vi "Stop HTTP.vi"(8 "error in (no error)":errorcluster, 11 "Vecto in":refnum<class "Vecto.lvclass">) -> (0 "error out":errorcluster, 3 "Vecto out":refnum<class "Vecto.lvclass">)   [LabVIEW 2020, in "Vecto.lvlib" / "Vecto.lvclass"]
uses:
  Vecto.lvclass
  Vecto.lvclass/Vecto.ctl
  lv-http-server/HTTP Server/Server/Server.lvclass
  VectoService/VectoInfo.lvclass
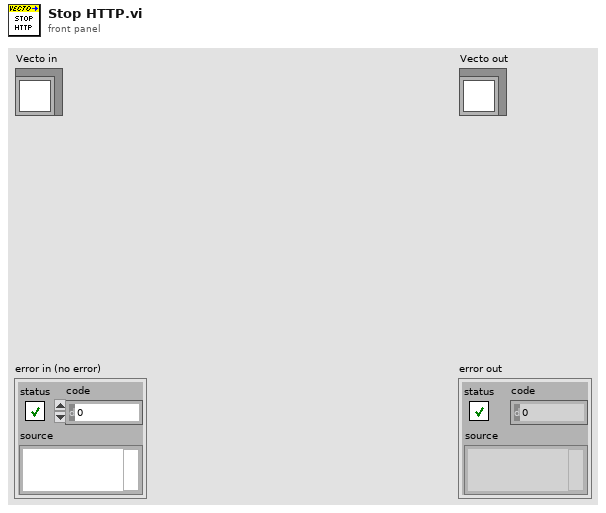
[diagram p1: front panel]
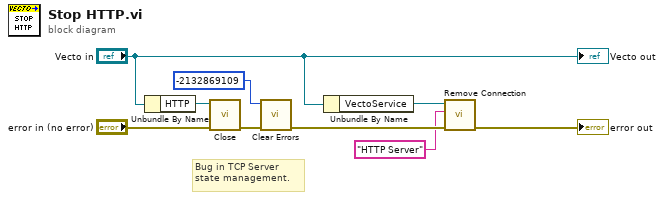
[diagram p0: block diagram]
diagram:
  # "Bug in TCP Server state management."
  n1 = Unbundle By Name("Vecto in") -> ("HTTP"=w8:refnum<class "Server.lvclass">)
  n2 = call "Close.vi"("error in (no error)"="error in (no error)", "Server in"=w8) -> ("error out"=w6:errorcluster)  [unwired: 8 in, 1 out]
  n3 = call <vilib>:"Clear Errors.vi"("error in (no error)"=w6, "specific error code to clear (0: all)"=-2132869109) -> ("error out"=w9:errorcluster)  [unwired: 4 in, 1 out]
  n4 = Unbundle By Name("Vecto in") -> ("VectoService"=w3:refnum<class "VectoInfo.lvclass">)
  n5 = call "Remove Connection.vi"("error in (no error)"=w9, "Connection Name"="HTTP Server", "VectoService in"=w3) -> ("error out"=→"error out":errorcluster)  [unwired: 7 in, 1 out]
  "Vecto out" <- "Vecto in"
